vi "RL env test - SAC.vi"() -> ()   [LabVIEW 2024]
uses:
  <vilib>/express/express arith-compare/Formula/XNode/ExpressFormulaBlockNode.xnode
  <vilib>/Analysis/NI_AALBase.lvlib
  <vilib>/measure/NI_MABase.lvlib
panel:
  out "total step":i32
  in  "幅值 2":dbl=1.0
  out "P":dbl(graph)=0.010526704867227326
  out "I":dbl(graph)=1.1597992766160083e-129
  out "start value":dbl[](array[numeric])=[-0.9724784126247488, -0.972476948667373, -0.9724754846716054, -0.9724740206374459, -0.9724725565648947, -0.9724710924539519, -0.9724696283046174, -0.9724681641168914, -0.9724666998907738, -0.9724652356262649, -0.9724637713233645, -0.9724623069820728, -0.9724608426023899, -0.9724593781843156, -0.9724579137278503, -0.9724564492329938, -0.9724549846997463, -0.9724535201281078, -0.9724520555180785, -0.9724505908696581, -0.9724491261828471, -0.9724476614576453, -0.9724461966940527, -0.9724447318920696, -0.9724432670516958, -0.9724418021729316, -0.9724403372557768, -0.9724388723002317, -0.9724374073062962, -0.9724359422739705, -0.9724344772032545, -0.9724330120941482, -0.972431546946652, -0.9724300817607656, -0.9724286165364893, -0.972427151273823, -0.9724256859727668, -0.9724242206333208, -0.972422755255485, -0.9724212898392596, -0.9724198243846445, -0.9724183588916397, -0.9724168933602455, -0.9724154277904618, -0.9724139621822886, -0.972412496535726, -0.9724110308507742, -0.972409565127433, -0.9724080993657028, -0.9724066335655833, -0.9724051677270749, -0.9724037018501773, -0.9724022359348908, -0.9724007699812155, -0.9723993039891512, -0.9723978379586983, -0.9723963718898565, -0.9723949057826261, -0.9723934396370071, -0.9723919734529995, -0.9723905072306035, -0.9723890409698189, -0.9723875746706461, -0.9723861083330848, -0.9723846419571354, -0.9723831755427976, -0.9723817090900718, -0.9723802425989578, -0.972378776069456, -0.972377309501566, -0.9723758428952882, -0.9723743762506224, -0.972372909567569, -0.9723714428461276, -0.9723699760862988, -0.9723685092880822, -0.9723670424514781, -0.9723655755764864, -0.9723641086631073, -0.9723626417113408, -0.972361174721187, -0.9723597076926458, -0.9723582406257175, -0.972356773520402, -0.9723553063766994, -0.9723538391946097, -0.9723523719741332, -0.9723509047152695, -0.9723494374180192, -0.9723479700823818, -0.9723465027083579, -0.9723450352959471, -0.9723435678451497, -0.9723421003559657, -0.9723406328283953, -0.9723391652624382, -0.972337697658095, -0.9723362300153652, -0.9723347623342492, -0.9723332946147469, -0.9723318268568585, -0.972330359060584, -0.9723288912259233, -0.9723274233528767, -0.9723259554414441, -0.9723244874916256, -0.9723230195034213, -0.9723215514768312, -0.9723200834118554, -0.972318615308494, -0.9723171471667469, -0.9723156789866143, -0.9723142107680962, -0.9723127425111927, -0.9723112742159038, -0.9723098058822296, -0.9723083375101702, -0.9723068690997255, -0.9723054006508958, -0.9723039321636809, -0.972302463638081, -0.9723009950740963, -0.9722995264717265, -0.972298057830972, -0.9722965891518325, -0.9722951204343085, -0.9722936516783997, -0.9722921828841063, -0.9722907140514283, -0.972289245180366, -0.972287776270919, -0.9722863073230879, -0.9722848383368722, -0.9722833693122724, -0.9722819002492883, -0.9722804311479202, -0.9722789620081678, -0.9722774928300315, -0.9722760236135111, -0.972274554358607, -0.9722730850653187, -0.972271615733647, -0.9722701463635912, -0.972268676955152, -0.972267207508329, -0.9722657380231224, -0.9722642684995324, -0.9722627989375588, -0.972261329337202, -0.9722598596984617, -0.9722583900213382, -0.9722569203058314, -0.9722554505519415, -0.9722539807596685, -0.9722525109290124, -0.9722510410599734, -0.9722495711525514, -0.9722481012067465, -0.9722466312225588, -0.9722451611999884, -0.9722436911390353, -0.9722422210396995, -0.9722407509019811, -0.9722392807258802, -0.9722378105113969, -0.972236340258531, -0.972234869967283, -0.9722333996376524, -0.97223192926964, -0.972230458863245, -0.9722289884184682, -0.972227517935309, -0.9722260474137682, -0.972224576853845, -0.9722231062555403, -0.9722216356188534, -0.9722201649437852, -0.9722186942303348, -0.9722172234785031, -0.9722157526882895, -0.9722142818596947, -0.9722128109927182, -0.9722113400873604, -0.9722098691436211, -0.9722083981615006, -0.9722069271409988, -0.9722054560821158, -0.9722039849848517, -0.9722025138492065, -0.9722010426751804, -0.9721995714627731, -0.9721981002119852, -0.9721966289228162, -0.9721951575952665, -0.9721936862293361, -0.972192214825025, -0.9721907433823334, -0.9721892719012611, -0.9721878003818084, -0.9721863288239753, -0.9721848572277617, -0.9721833855931679, -0.9721819139201937, -0.9721804422088394, -0.9721789704591048, -0.9721774986709903, -0.9721760268444957, -0.9721745549796211, -0.9721730830763666, -0.9721716111347323, -0.9721701391547182, -0.9721686671363242, -0.9721671950795507, -0.9721657229843975, -0.9721642508508648, -0.9721627786789525, -0.9721613064686608, -0.9721598342199897, -0.9721583619329394, -0.9721568896075097, -0.9721554172437008, -0.9721539448415127, -0.9721524724009456, -0.9721509999219994, -0.9721495274046742, -0.97214805484897, -0.9721465822548871, -0.9721451096224253, -0.9721436369515848, -0.9721421642423655, -0.9721406914947677, -0.9721392187087913, -0.9721377458844362, -0.9721362730217029, -0.972134800120591, -0.9721333271811009, -0.9721318542032323, -0.9721303811869858, -0.9721289081323609, -0.972127435039358, -0.9721259619079768, -0.9721244887382179, -0.9721230155300808, -0.9721215422835661, -0.9721200689986734, -0.972118595675403, -0.9721171223137549, -0.9721156489137291, -0.9721141754753259, -0.9721127019985449, -0.9721112284833866, -0.9721097549298509, -0.9721082813379377, -0.9721068077076473, -0.9721053340389797, -0.9721038603319349, -0.9721023865865129, -0.9721009128027139, -0.9720994389805379, -0.9720979651199849, -0.972096491221055, -0.9720950172837484, -0.9720935433080649, -0.9720920692940047, -0.9720905952415678, -0.9720891211507544, -0.9720876470215645, -0.972086172853998, -0.9720846986480551, -0.9720832244037358, -0.9720817501210404, -0.9720802757999685, -0.9720788014405206, -0.9720773270426963, -0.9720758526064963, -0.9720743781319199, -0.9720729036189679, -0.9720714290676397, -0.972069954477936, -0.972068479849856, -0.9720670051834008, -0.9720655304785695, -0.972064055735363, -0.9720625809537805, -0.972061106133823, -0.9720596312754896, -0.9720581563787812, -0.9720566814436972, -0.9720552064702382, -0.9720537314584037, -0.9720522564081945, -0.9720507813196096, -0.9720493061926503, -0.9720478310273155, -0.9720463558236063, -0.9720448805815217, -0.9720434053010629, -0.9720419299822287, -0.9720404546250205, -0.972038979229437, -0.9720375037954797, -0.9720360283231472, -0.9720345528124409, -0.9720330772633595, -0.9720316016759045, -0.9720301260500745, -0.972028650385871, -0.9720271746832927, -0.9720256989423409, -0.9720242231630145, -0.9720227473453147, -0.9720212714892403, -0.9720197955947928, -0.9720183196619707, -0.9720168436907757, -0.9720153676812061, -0.9720138916332638, -0.9720124155469471, -0.9720109394222577, -0.9720094632591939, -0.9720079870577577, -0.9720065108179472, -0.9720050345397644, -0.9720035582232074, -0.9720020818682782, -0.9720006054749749, -0.9719991290432995, -0.9719976525732502, -0.971996176064829, -0.9719946995180339, -0.9719932229328669, -0.9719917463093263, -0.9719902696474139, -0.9719887929471279, -0.9719873162084702, -0.9719858394314392, -0.9719843626160365, -0.9719828857622607, -0.9719814088701132, -0.9719799319395928, -0.9719784549707007, -0.9719769779634359, -0.9719755009177995, -0.9719740238337905, -0.9719725467114101, -0.9719710695506572, -0.9719695923515329, -0.9719681151140364, -0.9719666378381685, -0.9719651605239285, -0.9719636831713173, -0.971962205780334, -0.9719607283509797, -0.9719592508832534, -0.9719577733771562, -0.9719562958326872, -0.9719548182498473, -0.9719533406286357, -0.9719518629690534, -0.9719503852710996, -0.9719489075347751, -0.9719474297600792, -0.9719459519470128, -0.971944474095575, -0.971942996205767, -0.9719415182775876, -0.971940040311038, -0.9719385623061172, -0.9719370842628263, -0.9719356061811645, -0.9719341280611326, -0.9719326499027298, -0.9719311717059571, -0.9719296934708136, -0.9719282151973004, -0.9719267368854165, -0.971925258535163, -0.9719237801465389, -0.9719223017195453, -0.9719208232541813, -0.9719193447504477, -0.971917866208344, -0.9719163876278708, -0.9719149090090276, -0.971913430351815, -0.9719119516562326, -0.9719104729222808, -0.9719089941499593, -0.9719075153392687, -0.9719060364902085, -0.971904557602779, -0.9719030786769803, -0.9719015997128124, -0.9719001207102754, -0.9718986416693692, -0.9718971625900942, -0.9718956834724499, -0.971894204316437, -0.971892725122055, -0.9718912458893045, -0.971889766618185, -0.9718882873086971, -0.9718868079608404, -0.9718853285746153, -0.9718838491500215, -0.9718823696870594, -0.9718808901857288, -0.9718794106460301, -0.9718779310679628, -0.9718764514515277, -0.9718749717967241, -0.9718734921035527, -0.971872012372013, -0.9718705326021055, -0.9718690527938301, -0.9718675729471868, -0.9718660930621756, -0.9718646131387969, -0.9718631331770503, -0.9718616531769363, -0.9718601731384545, -0.9718586930616054, -0.9718572129463887, -0.9718557327928048, -0.9718542526008533, -0.9718527723705349, -0.971851292101849, -0.9718498117947961, -0.9718483314493759, -0.971846851065589, -0.9718453706434347, -0.971843890182914, -0.9718424096840259, -0.9718409291467714, -0.9718394485711499, -0.971837967957162, -0.9718364873048071, -0.9718350066140861, -0.971833525884998, -0.9718320451175441, -0.9718305643117232, -0.9718290834675365, -0.971827602584983, -0.9718261216640638, -0.971824640704778, -0.9718231597071265, -0.9718216786711086, -0.9718201975967251, -0.9718187164839752, -0.97181723533286, -0.9718157541433784, -0.9718142729155317, -0.9718127916493186, -0.9718113103447406, -0.9718098290017962, -0.9718083476204872, -0.9718068662008119, -0.9718053847427719, -0.9718039032463659, -0.9718024217115953, -0.9718009401384589, -0.9717994585269578, -0.9717979768770911, -0.9717964951888599, -0.9717950134622632, -0.9717935316973021, -0.9717920498939755, -0.9717905680522848, -0.9717890861722286, -0.9717876042538085, -0.9717861222970229, -0.9717846403018736, -0.9717831582683589, -0.9717816761964806, -0.9717801940862371, -0.97177871193763, -0.9717772297506578, -0.9717757475253223, -0.9717742652616217, -0.9717727829595578, -0.9717713006191291, -0.9717698182403373, -0.9717683358231806, -0.9717668533676609, -0.9717653708737766, -0.9717638883415293, -0.9717624057709174, -0.9717609231619428, -0.9717594405146038, -0.9717579578289021, -0.9717564751048361, -0.9717549923424075, -0.9717535095416148, -0.9717520267024594, -0.9717505438249402, -0.9717490609090584, -0.9717475779548129, -0.971746094962205, -0.9717446119312335, -0.9717431288618996, -0.9717416457542023, -0.9717401626081427, -0.9717386794237198, -0.9717371962009347, -0.9717357129397864, -0.9717342296402761, -0.9717327463024028, -0.9717312629261674, -0.9717297795115692, -0.9717282960586091, -0.9717268125672862, -0.9717253290376016, -0.9717238454695543, -0.9717223618631453, -0.9717208782183738, -0.9717193945352408, -0.9717179108137454, -0.9717164270538886, -0.9717149432556694, -0.971713459419089, -0.9717119755441463, -0.9717104916308427, -0.9717090076791767, -0.9717075236891499, -0.9717060396607609, -0.9717045555940113, -0.9717030714888995, -0.9717015873454271, -0.9717001031635928, -0.971698618943398, -0.9716971346848414, -0.9716956503879245, -0.9716941660526458, -0.9716926816790069, -0.9716911972670064, -0.9716897128166457, -0.9716882283279236, -0.9716867438008415, -0.971685259235398, -0.9716837746315946, -0.97168228998943, -0.9716808053089055, -0.97167932059002, -0.9716778358327749, -0.9716763510371687, -0.971674866203203, -0.9716733813308763, -0.9716718964201904, -0.9716704114711435, -0.9716689264837375, -0.9716674414579707, -0.9716659563938448, -0.9716644712913582, -0.9716629861505127, -0.9716615009713067, -0.9716600157537418, -0.9716585304978165, -0.9716570452035325, -0.9716555598708881, -0.9716540744998852, -0.9716525890905221, -0.9716511036428004, -0.9716496181567188, -0.9716481326322787, -0.9716466470694788, -0.9716451614683205, -0.9716436758288024, -0.9716421901509261, -0.9716407044346902, -0.9716392186800963, -0.9716377328871427, -0.9716362470558313, -0.9716347611861603, -0.9716332752781316, -0.9716317893317435, -0.9716303033469977, -0.9716288173238928, -0.9716273312624302, -0.9716258451626086, -0.9716243590244295, -0.9716228728478914, -0.9716213866329959, -0.9716199003797417, -0.9716184140881301, -0.9716169277581599, -0.9716154413898325, -0.9716139549831465, -0.9716124685381035, -0.971610982054702, -0.9716094955329435, -0.9716080089728268, -0.9716065223743532, -0.9716050357375214, -0.9716035490623329, -0.9716020623487863, -0.9716005755968832, -0.9715990888066219, -0.9715976019780044, -0.9715961151110288, -0.9715946282056971, -0.9715931412620074, -0.9715916542799616, -0.971590167259558, -0.9715886802007986, -0.9715871931036814, -0.9715857059682085, -0.9715842187943778, -0.9715827315821917, -0.9715812443316478, -0.9715797570427487, -0.9715782697154919, -0.97157678234988, -0.9715752949459104, -0.971573807503586, -0.9715723200229041, -0.9715708325038672, -0.9715693449464731, -0.9715678573507242, -0.971566369716618, -0.9715648820441573, -0.9715633943333394, -0.971561906584167, -0.9715604187966376, -0.9715589309707537, -0.971557443106513, -0.9715559552039181, -0.9715544672629663, -0.9715529792836605, -0.9715514912659979, -0.9715500032099813, -0.9715485151156082, -0.9715470269828812, -0.9715455388117977, -0.9715440506023605, -0.9715425623545669, -0.9715410740684197, -0.9715395857439163, -0.9715380973810593, -0.9715366089798463, -0.9715351205402798, -0.9715336320623573, -0.9715321435460815, -0.97153065499145, -0.9715291663984651, -0.9715276777671246, -0.9715261890974309, -0.9715247003893817, -0.9715232116429795, -0.9715217228582218, -0.9715202340351112, -0.9715187451736453, -0.9715172562738267, -0.9715157673356528, -0.9715142783591263, -0.9715127893442447, -0.9715113002910105, -0.9715098111994214, -0.9715083220694798, -0.9715068329011833, -0.9715053436945347, -0.9715038544495311, -0.9715023651661755, -0.9715008758444652, -0.9714993864844028, -0.971497897085986, -0.9714964076492172, -0.971494918174094, -0.9714934286606189, -0.9714919391087896, -0.9714904495186086, -0.9714889598900734, -0.9714874702231867, -0.9714859805179459, -0.9714844907743536, -0.9714830009924074, -0.9714815111721098, -0.9714800213134585, -0.9714785314164558, -0.9714770414810995, -0.9714755515073921, -0.971474061495331, -0.971472571444919, -0.9714710813561536, -0.9714695912290372, -0.9714681010635675, -0.9714666108597471, -0.9714651206175734, -0.9714636303370491, -0.9714621400181717, -0.9714606496609437, -0.9714591592653627, -0.9714576688314314, -0.9714561783591472, -0.9714546878485126, -0.9714531972995254, -0.971451706712188, -0.9714502160864978, -0.9714487254224577, -0.971447234720065, -0.9714457439793225, -0.9714442532002274, -0.9714427623827827, -0.9714412715269855, -0.9714397806328388, -0.9714382897003396, -0.9714367987294912, -0.9714353077202904, -0.9714338166727405, -0.9714323255868383, -0.9714308344625872, -0.9714293432999838, -0.9714278520990316, -0.9714263608597272, -0.9714248695820743, -0.9714233782660692, -0.9714218869117157, -0.9714203955190102, -0.9714189040879564, -0.9714174126185505, -0.9714159211107967, -0.9714144295646908, -0.9714129379802371, -0.9714114463574315, -0.9714099546962781, -0.9714084629967731, -0.9714069712589203, -0.9714054794827159, -0.9714039876681639, -0.9714024958152606, -0.9714010039240096, -0.9713995119944075, -0.9713980200264579, -0.9713965280201572, -0.9713950359755091, -0.9713935438925101, -0.9713920517711638, -0.9713905596114667, -0.9713890674134225, -0.9713875751770275, -0.9713860829022855, -0.9713845905891928, -0.9713830982377533, -0.9713816058479632, -0.9713801134198264, -0.9713786209533392, -0.9713771284485054, -0.9713756359053212, -0.9713741433237907, -0.9713726507039097, -0.9713711580456826, -0.9713696653491052, -0.9713681726141818, -0.9713666798409082, -0.9713651870292888, -0.9713636941793191, -0.9713622012910038, -0.9713607083643384, -0.9713592153993275, -0.9713577223959665, -0.9713562293542602, -0.971354736274204, -0.9713532431558026, -0.9713517499990513, -0.971350256803955, -0.9713487635705088, -0.9713472702987179, -0.9713457769885772, -0.9713442836400918, -0.9713427902532568, -0.9713412968280771, -0.971339803364548, -0.9713383098626744, -0.9713368163224514, -0.9713353227438841, -0.9713338291269674, -0.9713323354717066, -0.9713308417780966, -0.9713293480461425, -0.9713278542758393, -0.9713263604671921, -0.9713248666201961, -0.9713233727348561, -0.9713218788111675, -0.9713203848491349, -0.9713188908487538, -0.9713173968100288, -0.9713159027329555, -0.9713144086175385, -0.9713129144637732, -0.9713114202716644, -0.9713099260412074, -0.9713084317724069, -0.9713069374652584, -0.9713054431197665, -0.9713039487359268, -0.9713024543137437, -0.9713009598532131, -0.9712994653543391, -0.9712979708171176, -0.9712964762415529, -0.9712949816276408, -0.9712934869753858, -0.9712919922847834, -0.9712904975558381, -0.9712890027885456, -0.9712875079829103, -0.971286013138928, -0.971284518256603, -0.9712830233359311, -0.9712815283769166, -0.9712800333795553, -0.9712785383438516, -0.9712770432698011, -0.9712755481574084, -0.971274053006669, -0.9712725578175875, -0.9712710625901595, -0.9712695673243894, -0.971268072020273, -0.9712665766778146, -0.97126508129701, -0.9712635858778634, -0.9712620904203709, -0.9712605949245365, -0.9712590993903563, -0.9712576038178343, -0.9712561082069665, -0.9712546125577572, -0.9712531168702022, -0.9712516211443057, -0.9712501253800637, -0.9712486295774804, -0.9712471337365516, -0.9712456378572816, -0.9712441419396662, -0.9712426459837098, -0.9712411499894081, -0.9712396539567655, -0.9712381578857778, -0.9712366617764492, -0.9712351656287758, -0.9712336694427613, -0.9712321732184024, -0.9712306769557024, -0.9712291806546581, -0.971227684315273, -0.9712261879375435, -0.9712246915214733, -0.9712231950670589, -0.971221698574304, -0.9712202020432049, -0.9712187054737655, -0.9712172088659821, -0.9712157122198584, -0.9712142155353907, -0.971212718812583, -0.9712112220514313, -0.9712097252519398, -0.9712082284141044, -0.9712067315379294, -0.9712052346234105, -0.971203737670552, -0.9712022406793499, -0.9712007436498084, -0.9711992465819232, -0.9711977494756988, -0.9711962523311309, -0.9711947551482238, -0.9711932579269735, -0.971191760667384, -0.9711902633694514, -0.9711887660331797, -0.971187268658565, -0.9711857712456115, -0.9711842737943148, -0.9711827763046796, -0.9711812787767015, -0.9711797812103848, -0.9711782836057253, -0.9711767859627275, -0.9711752882813869, -0.971173790561708, -0.9711722928036866, -0.971170795007327, -0.9711692971726248, -0.9711677992995847, -0.9711663013882021, -0.9711648034384818, -0.9711633054504191, -0.9711618074240187, -0.971160309359276, -0.9711588112561959, -0.9711573131147735, -0.9711558149350138, -0.971154316716912, -0.971152818460473, -0.971151320165692, -0.9711498218325738, -0.9711483234611138, -0.9711468250513168, -0.971145326603178, -0.9711438281167024, -0.9711423295918851, -0.9711408310287312, -0.9711393324272355, -0.9711378337874035, -0.9711363351092298, -0.9711348363927199, -0.9711333376378684, -0.9711318388446808, -0.9711303400131517, -0.9711288411432867, -0.9711273422350802, -0.9711258432885381, -0.9711243443036546, -0.9711228452804355, -0.9711213462188751, -0.9711198471189793, -0.9711183479807423, -0.9711168488041699, -0.9711153495892566, -0.9711138503360079, -0.9711123510444185, -0.9711108517144939, -0.9711093523462285, -0.9711078529396281, -0.9711063534946871, -0.9711048540114111, -0.9711033544897947, -0.9711018549298434, -0.9711003553315518, -0.9710988556949254, -0.971097356019959, -0.9710958563066576, -0.9710943565550165, -0.9710928567650405, -0.971091356936725, -0.9710898570700747, -0.9710883571650849, -0.9710868572217604, -0.9710853572400966, -0.9710838572200982, -0.9710823571617607, -0.9710808570650886, -0.9710793569300776, -0.9710778567567321, -0.9710763565450479, -0.9710748562950291, -0.9710733560066719, -0.9710718556799801, -0.9710703553149501, -0.9710688549115856, -0.971067354469883, -0.971065853989846, -0.9710643534714711, -0.9710628529147619, -0.9710613523197149, -0.9710598516863337, -0.9710583510146148, -0.9710568503045618, -0.9710553495561713, -0.9710538487694468, -0.971052347944385, -0.9710508470809891, -0.9710493461792562, -0.9710478452391892, -0.9710463442607854, -0.9710448432440476, -0.9710433421889731, -0.9710418410955648, -0.9710403399638199, -0.9710388387937412, -0.9710373375853261, -0.9710358363385773, -0.9710343350534921, -0.9710328337300734, -0.9710313323683186, -0.9710298309682303, -0.971028329529806, -0.9710268280530482, -0.9710253265379547, -0.9710238249845278, -0.9710223233927653, -0.9710208217626694, -0.9710193200942381, -0.9710178183874735, -0.9710163166423736, -0.9710148148589407, -0.9710133130371725, -0.9710118111770714, -0.9710103092786351, -0.971008807341866, -0.9710073053667618, -0.9710058033533251, -0.9710043013015532, -0.971002799211449, -0.9710012970830099, -0.9709997949162384, -0.9709982927111321, -0.9709967904676936]
  out "I":dbl=1.1597992766160083e-129
  out "P":dbl=0.010526704867227326
  out "ZVolt":dbl(graph)=0.314
  out "largest reward episode":picture
  out "initialized array":dbl[](array[numeric])
  out "ep reward":dbl(graph)=11.830070995768676
  out "loss_c":dbl(graph)=1731497.5
  out "loss_a":dbl(graph)=6725.31298828125
  out "max ep reward":dbl=24543.99785734303
  out "batch_size":i32=256
  in  "base batch number":i32=256
  out "ep reward":dbl=3677.849231856129
  out "PIDoutput":dbl=0.0008497199147603398
  out "Reward":dbl=4.912643239900043
  out "errorsum":dbl=-0.005069024381114479
  out "ZVolt":dbl=0.129
  out "return value":dbl[](array[numeric])=[0.128, -0.005028664176972831, 0.0008485916053116275, 4.912763807403283, 5000.08984375, 122631.6953125, 0.01052668650438312, 1.663726715006467e-129, 30902.0]
  out "loss_c":dbl=23912.59765625
  out "loss_a":dbl=4978.1279296875
  out "ep loop":i32=506
  out "topo":dbl[][](array[numeric])
  in  "扫描像素":i32=500
  in  "deflection setpoint\nV":dbl=0.5 caption="defl setpoint\n/V" format="%.2f"
  in  "spring constant\nN/m":dbl=2.34
  in  "invOLS\nm/V":dbl=1e-07
  in  "noise amp":dbl caption="noise 幅值" format="%0.2f"
  out "tem topo":dbl[](array[numeric])=[187.7613450258975, 187.61388643049506, 187.4625946204324, 187.30747590277633, 187.14853587042907, 186.98578082132366, 186.81921706928887, 186.64885137876908, 186.4746905808606, 186.29674199265563, 186.1150123695872, 185.92950817277307, 185.74023679128615, 185.5472059277571, 185.3504235460163, 185.14989781279343, 184.94563633899963, 184.7376469430854, 184.52593768641884, 184.3105160636524, 184.09139078628462, 183.86857162664072, 183.64206782984775, 183.41188762880165, 183.17803969715476, 182.940533253404, 182.6993776738212, 182.45458275299467, 182.2061581201141, 181.9541137790551, 181.69845902351616, 181.4392040047092, 181.17635923335035, 180.9099353647009, 180.63994279021992, 180.36639272167008, 180.0892956631369, 179.80866218898547, 179.52450272102482, 179.23682835570867, 178.9456510293229, 178.6509823562041, 178.35283451751783, 178.05121924067203, 177.74614789904152, 177.43763209086856, 177.1256831579414, 176.81031438615872, 176.49153920701886, 176.1693704250344, 175.8438197839498, 175.5148992710352, 175.1826220036406, 174.84700179662502, 174.50805226675456, 174.1657866700021, 173.82021882777377, 173.4713618312618, 173.11922905760952, 172.76383369071877, 172.40519035359426, 172.04331373418668, 171.67821862608477, 171.309919247784, 170.93842996746667, 170.56376459454503, 170.1859381629234, 169.80496661154504, 169.42086450264173, 169.0336461495204, 168.64332644908936, 168.24992153572245, 167.8534472210812, 167.45391914002545, 167.05135290786737, 166.64576477592976, 166.23717056004534, 165.8255864580667, 165.41102824418462, 164.993512051037, 164.5730539824388, 164.14967149000674, 163.72338154946098, 163.29420163843847, 162.8621478997749, 162.42723600545892, 161.98948326866116, 161.54890821264763, 161.10552891654612, 160.65936182203373, 160.2104244383099, 159.75873339582176, 159.30430783151849, 158.84716617980712, 158.38732582179352, 157.92480465368322, 157.45962095462795, 156.9917931204645, 156.52134079311634, 156.04828181301244, 155.5726339452858, 155.09441638968062, 154.6136472489628, 154.13034603381615, 153.64453342334664, 153.15622823962474, 152.6654487644259, 152.17221427862043, 151.67654406165875, 151.17845773475776, 150.6779754198373, 150.1751166395368, 149.6699009678266, 149.16234857689454, 148.65247965734684, 148.14031472217746, 147.6258735036707, 147.10917499961235, 146.59023960513701, 146.06908936048072, 145.54574534752848, 145.0202280189793, 144.49255697285886, 143.9627528409633, 143.43083662447464, 142.89683103403888, 142.36075609849416, 141.8226322377577, 141.28248084096668, 140.7403228358143, 140.19618147026964, 139.65007719448658, 139.10203138144058, 138.5520648385552, 138.0001998189378, 137.44645916616463, 136.8908646299422, 136.33343835957476, 135.77420029905568, 135.2131729773161, 134.65037927199438, 134.085842517716, 133.51958398463665, 132.95162590146327, 132.38198951126483, 131.81069772747327, 131.23777582486153, 130.66324602136686, 130.08712810940673, 129.50944270227356, 128.9302148852338, 128.34946995048892, 127.76723132900268, 127.1835223957668, 126.59836313273254, 126.0117743805774, 125.42378171891849, 124.83440802553078, 124.24367865056477, 123.65161705267003, 123.05824537033818, 122.46358737016546, 121.8676660763033, 121.27050397839896, 120.67212509303626, 120.07255452365224, 119.47181429525949, 118.86992771340098, 118.26691945109958, 117.66281486922844, 117.05763699983594, 116.45140914898187, 115.84415486761131, 115.23589739677422, 114.62666129469993, 114.01647170371834, 113.4053523678418, 112.79332761724639, 112.18042094737417, 111.56665539163178, 110.95205657012772, 110.33664908843807, 109.7204567805789, 109.10350337562569, 108.48581429969163, 107.86741457937245, 107.24832916589155, 106.62858082996027, 106.00819263635799, 105.38718869341413, 104.76559399003862, 104.1434364037364, 103.52074069435302, 102.89752945766561, 102.27382523581976, 101.64965224143607, 101.0250378083464, 100.4000075640133, 99.77458579919268, 99.1487949153723, 98.52265906971381, 97.89620440697074, 97.26945584154277, 96.64244000241739, 96.01518209293741, 95.38770529956422, 94.76003198981391, 94.13218671610107, 93.50419571582589, 92.87608519661319, 92.24788071347997, 91.61960554934515, 90.99128322185149, 90.36293885140294, 89.73459833622178, 89.10628770918771, 88.47803030643058, 87.84985008435751, 87.22177373506835, 86.59382458272312, 85.96602876753649, 85.33841005320626, 84.71099133420107, 84.08379740659025, 83.45685581207407, 82.83019160660528, 82.20382991407092, 81.57779526064273, 80.95210936674015, 80.32679554916554, 79.70188178789725, 79.07739412234078, 78.45335970976134, 77.82979964411959, 77.2067353165578, 76.5841915304312, 75.96219562894171, 75.34077282899595, 74.71994845171014, 74.0997464577927, 73.48018780517437, 72.8612969192854, 72.24310150008678, 71.62562695271967, 71.00889694495794, 70.39293416106386, 69.77776243437484]
  in  "frequency 2":dbl=0.001
  in  "amplitude":dbl caption="幅值 1" format="%0.2p"
  in  "effective\nmodulus\nPa":dbl=1500000000.0
  in  "tip\nradius\nnm":dbl=1e-08
  in  "a0\nnm 2":dbl=4e-10
  in  "hamaker\nconstant":dbl=4.25e-19
  out "Fs":dbl=1000.0
  out "error":dbl(graph)=0.0806133634699095
  out "#s":dbl=1000.0
  in  "sampling info":cluster{"Fs":dbl, "#s":dbl}={"Fs"=1000.0, "#s"=1000.0} caption="采样信息" {"Fs" format="%.2p"}
  in  "frequency":dbl=0.01 caption="frequency 1" format="%0.2p"
  out "separation":dbl(graph)=-6.006813032198851e-09
  out "defl voltage":dbl(graph)=0.4193866365300905
  out "control signal":dbl(graph)=0.9638211864355544
  out "sample surface":dbl[][](graph)=[[76.39974719326271, 70.39293416106386]]
  out "done":bool
  out "step loop":i32=747
types:
  T1 = typedef "imagedata.ctl" = cluster{"image type":i32, "image depth":i32, "image":u8[], "mask":u8[], "colors":u32[], "Rectangle":cluster{"left":i16, "top":i16, "right":i16, "bottom":i16}}
  T2 = typedef "NI_Matrix.lvlib/RealMatrix.ctl" = dbl[][]
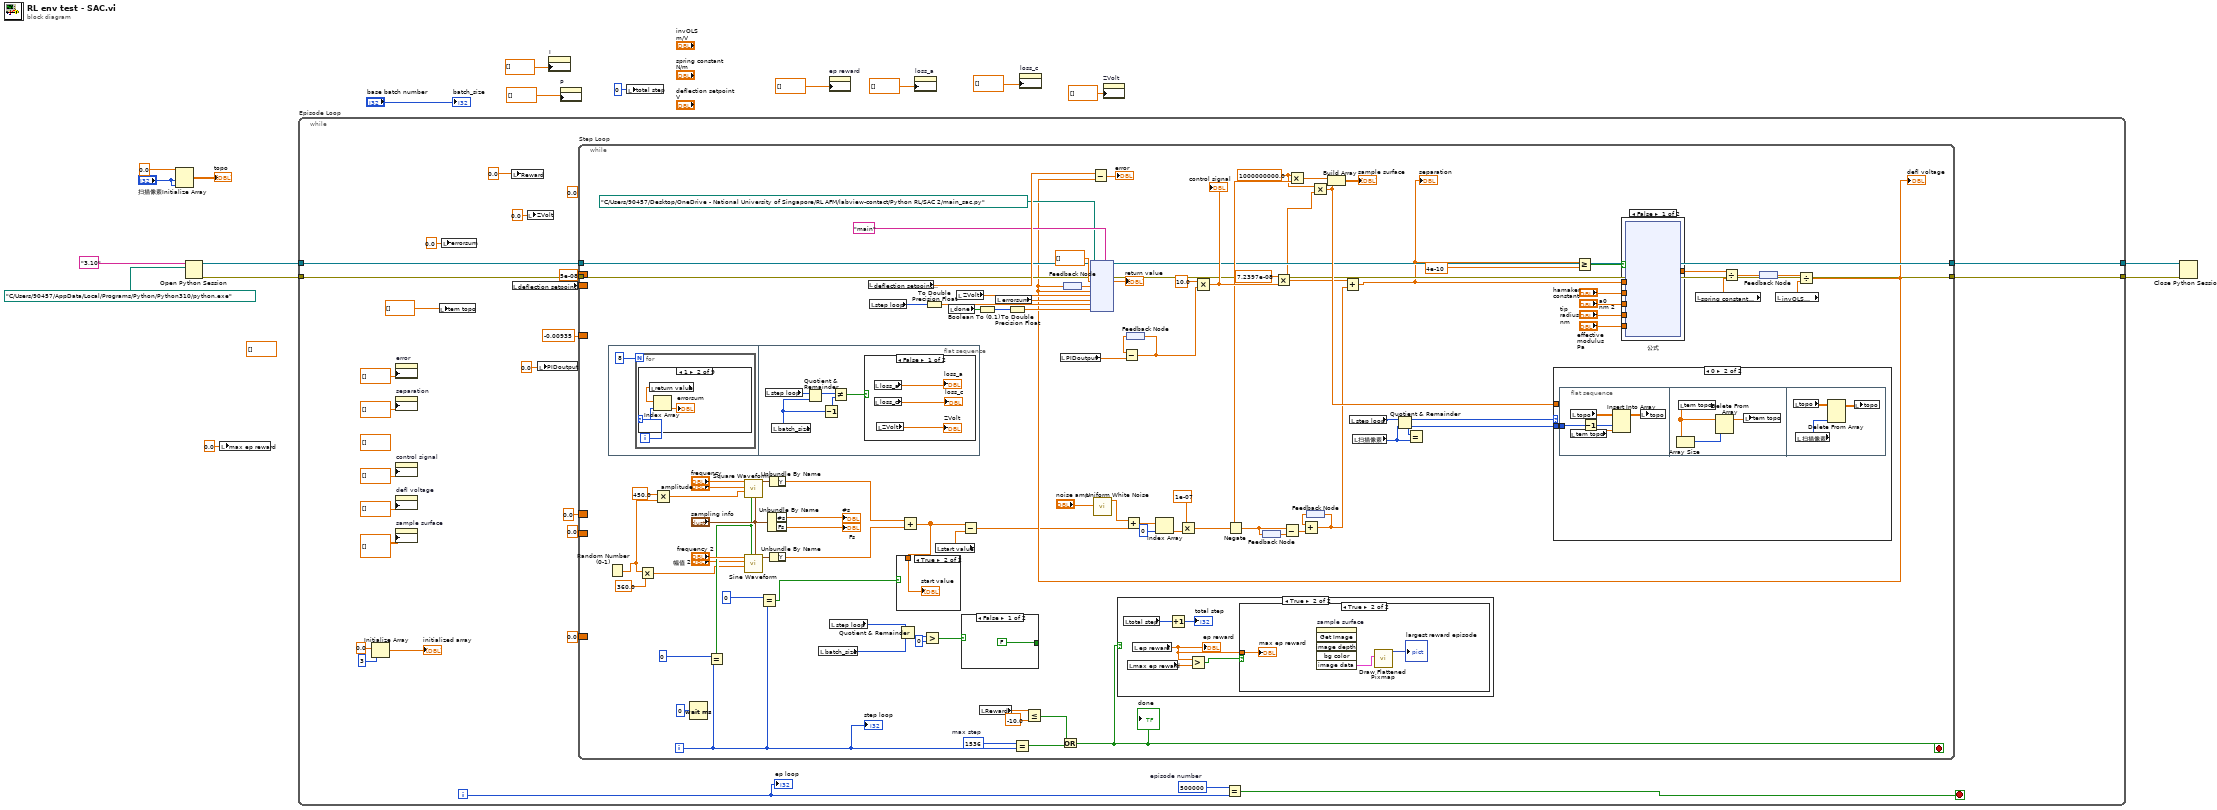
[diagram p0: block diagram]
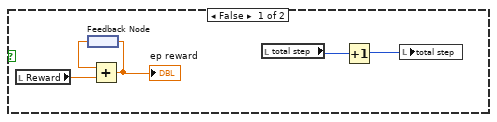
[diagram p3: hidden frame]
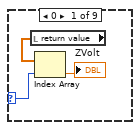
[diagram p5: hidden frame]
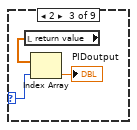
[diagram p6: hidden frame]
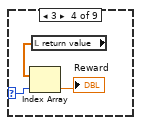
[diagram p7: hidden frame]
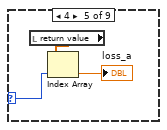
[diagram p8: hidden frame]
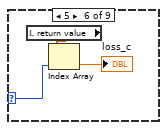
[diagram p9: hidden frame]
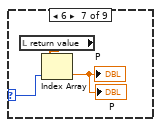
[diagram p10: hidden frame]
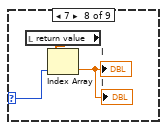
[diagram p11: hidden frame]
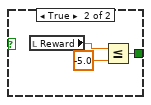
[diagram p14: hidden frame]
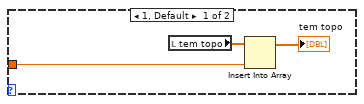
[diagram p15: hidden frame]
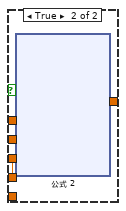
[diagram p16: hidden frame]
diagram:
  (unwired) dbl[] []
  n1 = Initialize Array(0.0 ("元素"), "扫描像素", "扫描像素") -> (→"topo":dbl[][])
  n2 = Open Python Session(python version="3.10" ("Python version"), python path=path "C:/Users/90457/AppData/Local/Programs/Python/Python310/python.exe" ("Python path")) -> (session out=w15:refnum<k35>, error out=w14:errorcluster)  [unwired: 1 in]
  n3 = local write "max ep reward"(0.0 ("max ep reward")) -> ()
  n4 = while "Episode Loop" {
    tunnel: w15 -> [w30]
    tunnel: w14 -> [w29]
    tunnel: [w28] -> w11
    tunnel: [w27] -> w10
    i -> [w40]
    stop <- w44 stop-if-true
    (unwired) 0.0
    (unwired) dbl[] [] ("History Data")
    w32 = 500000  # episode number
    n5 = Initialize Array(0.0 ("element"), 3 ("dimension size")) -> (→"initialized array":dbl[])
    n6 = property on="error" class="WFChart (strict)"("History Data"=dbl[] []) -> ()  [unwired: 2 in, 2 out]
    n7 = property on="separation" class="WFChart (strict)"("History Data"=dbl[] []) -> ()  [unwired: 2 in, 2 out]
    n8 = property on="control signal" class="WFChart (strict)"("History Data"=dbl[] []) -> ()  [unwired: 2 in, 2 out]
    n9 = property on="defl voltage" class="WFChart (strict)"("History Data"=dbl[] []) -> ()  [unwired: 2 in, 2 out]
    n10 = property on="sample surface" class="WFChart (strict)"("History Data"=dbl[][] []) -> ()  [unwired: 2 in, 2 out]
    n11 = local write "tem topo"(dbl[] [] ("History Data")) -> ()
    n12 = local write "errorsum"(0.0 ("errorsum")) -> ()
    n13 = local write "Reward"(0.0) -> ()
    n14 = local read "deflection setpoint\nV"() -> (w43:dbl)
    n15 = local write "ZVolt"(0.0 ("ZVolt")) -> ()
    n16 = local write "PIDoutput"(0.0 ("PIDoutput")) -> ()
    n17 = while "Step Loop" {
      tunnel: [w94] -> w28
      tunnel: [w68] -> w27
      border: w43 -> [_]
      border: 0.0 -> [_]
      border: 5e-08 -> [_]
      border: 0.0 -> [_]
      tunnel: w30 -> [w72]
      tunnel: w29 -> [w71]
      border: 0.0 -> [_]
      border: -0.00935 -> [_]
      i -> [w64]
      stop <- w73 stop-if-true
      w111 = 1000000000.0 ("x")
      w88 = 1536  # max step
      n18 = flat-sequence {
        frame #0 {
          n19 = for {
            N: 8 -> [_]
            i -> [w154]
            n20 = case shown="1" w154 {
              selector: w154 -> [w157 w160 w161 w166 w169 w172 w174 w177 _]
              frame 0 {
                n21 = local read "return value"() -> (w156:dbl[])
                n22 = Index Array(array=w156, index=w157) -> (element=→"ZVolt":dbl)
              }
              frame 1 {
                n23 = local read "return value"() -> (w159:dbl[])
                n24 = Index Array(array=w159, index=w160) -> (element=→"errorsum":dbl)
              }
              frame 2 {
                n25 = local read "return value"() -> (w163:dbl[])
                n26 = Index Array(array=w163, index=w161) -> (element=→"PIDoutput":dbl)
              }
              frame 3 {
                n27 = local read "return value"() -> (w165:dbl[])
                n28 = Index Array(array=w165, index=w166) -> (element=→"Reward":dbl)
              }
              frame 4 {
                n29 = local read "return value"() -> (w168:dbl[])
                n30 = Index Array(array=w168, index=w169) -> (element=→"loss_a":dbl)
              }
              frame 5 {
                n31 = local read "return value"() -> (w171:dbl[])
                n32 = Index Array(array=w171, index=w172) -> (element=→"loss_c":dbl)
              }
              frame 6 {
                n33 = local read "return value"() -> (w175:dbl[])
                n34 = Index Array(array=w175, index=w174) -> (element=→"P" →"P":dbl)
              }
              frame 7 {
                n35 = local read "return value"() -> (w178:dbl[])
                n36 = Index Array(array=w178, index=w177) -> (element=→"I" →"I":dbl)
              }
              frame 9, Default {
              }
            }
          }
        }
        frame #1 {
          n37 = local read "step loop"() -> (w181:i32)
          n38 = local read "batch_size"() -> (w179:i32)
          n39 = Quotient & Remainder(x=w181, y=w179) -> (x-y*floor(x/y)=w182:i32)  [unwired: 1 out]
          n40 = Decrement(x=w179) -> (x-1=w180:i32)
          n41 = Not Equal?(x=w182, y=w180) -> (x != y?=w183:bool)
          n42 = case shown="False" w183 {
            frame False {
              n43 = local read "loss_a"() -> (→"loss_a":dbl)
              n44 = local read "loss_c"() -> (→"loss_c":dbl)
              n45 = local read "ZVolt"() -> (→"ZVolt":dbl)
            }
            frame True {
            }
          }
        }
      }
      n46 = Random Number (0-1)() -> (number: 0 to 1=w46:dbl)
      n47 = Multiply(x=w46, y=360.0) -> (x*y=w53:dbl)
      n48 = Multiply(x=450.0, y=w46) -> (x*y=w47:dbl)
      n49 = Wait (ms)(milliseconds to wait=u32 0) -> ()  [unwired: 1 out]
      n50 = Equal?(x=0, y=w64) -> (x = y?=w86:bool)
      n51 = call <vilib>:"Square Waveform.vi"("sampling info"="sampling info", "reset signal"=w86, "phase"=w47, "amplitude"="amplitude", "frequency"="frequency") -> ("signal out"=w133:waveform(dbl))  [unwired: 5 in, 1 out]
      n52 = call <vilib>:"Sine Waveform.vi"("sampling info"="sampling info", "reset signal"=w86, "phase"=w53, "amplitude"="幅值 2", "frequency"="frequency 2") -> ("signal out"=w109:waveform(dbl))  [unwired: 5 in, 1 out]
      n53 = Equal?(x=0, y=w64) -> (x = y?=w66:bool)
      n54 = Unbundle By Name("sampling info") -> ("#s"=→"#s":dbl, "Fs"=→"Fs":dbl)
      n55 = Unbundle By Name(w133) -> ("Y"=w101:dbl[])
      n56 = Unbundle By Name(w109) -> ("Y"=w65:dbl[])
      n57 = local read "batch_size"() -> (w69:i32)
      n58 = local read "step loop"() -> (w84:i32)
      n59 = local read "deflection setpoint\nV"() -> (w100:dbl)
      n60 = local read "step loop"() -> (w89:i32)
      n61 = Quotient & Remainder(x=w84, y=w69) -> (floor(x/y)=w83:i32)  [unwired: 1 out]
      n62 = Add(x=w101, y=w65) -> (x+y=w50:dbl[])
      n63 = case shown="True" w66 {
        tunnel: w50 -> [_ w139]
        frame False {
        }
        frame True {
          "start value" <- w139
        }
      }
      n64 = Greater?(x=w83, y=0) -> (0:w81:bool)
      n65 = To Double Precision Float(number=w89) -> (double precision float=w79:dbl)
      n66 = local read "start value"() -> (w52:dbl[])
      n67 = local read "done"() -> (w91:bool)
      n68 = local read "ZVolt"() -> (w74:dbl)
      n69 = case shown="False" w81 {
        tunnel: [FALSE w188] -> _
        frame False {
        }
        frame True {
          n70 = local read "Reward"() -> (w189:dbl)
          n71 = Less Or Equal?(x=w189, y=-5.0) -> (x <= y?=w188:bool)
        }
      }
      n72 = Subtract(x=w50, y=w52) -> (x-y=w51:dbl[])
      n73 = Boolean To (0,1)(Boolean=w91) -> (0, 1=w93:i16)
      n74 = local read "Reward"() -> (w77:dbl)
      n75 = local read "errorsum"() -> (w75:dbl)
      n76 = To Double Precision Float(number=w93) -> (double precision float=w80:dbl)
      n77 = Equal?(x=w88, y=w64) -> (x = y?=w78:bool)
      n78 = Less Or Equal?(x=w77, y=-10.0) -> (x <= y?=w49:bool)
      n79 = local read "PIDoutput"() -> (w57:dbl)
      n80 = Or(x=w49, y=w78) -> (x .or. y?=w73:bool)
      "done" <- w73
      n81 = feedback #1 ("反馈节点")() -> (w95:dbl)
      n82 = call <vilib>:"Uniform White Noise.vi"("amplitude"="noise amp") -> ("uniform white noise"=w103:dbl[])  [unwired: 9 in, 1 out]
      n83 = case shown="True" w73 {
        frame False {
          n84 = local read "Reward"() -> (w144:dbl)
          n85 = feedback #2() -> (w142:dbl)
          n86 = Add(x=w142, y=w144) -> (x+y=w143:dbl)
          "ep reward" <- w143
          n87 = feedback-in #2(w143) -> ()
          n88 = local read "total step"() -> (w141:i32)
          n89 = Increment(x=w141) -> (x+1=w140:i32)
          n90 = local write "total step"(w140) -> ()
        }
        frame True {
          n91 = local read "total step"() -> (w146:i32)
          n92 = local read "max ep reward"() -> (w148:dbl)
          n93 = local read "ep reward"() -> (w147:dbl)
          "ep reward" <- w147
          n94 = Increment(x=w146) -> (x+1=→"total step":i32)
          n95 = Greater?(x=w147, y=w148) -> (0:w149:bool)
          n96 = case shown="True" w149 {
            tunnel: w147 -> [_ w152]
            frame False {
            }
            frame True {
              n97 = invoke on="sample surface" class="WFChart (strict)" method="Get Image"() -> ("image data"=w151:T1)  [unwired: 6 in, 5 out]
              n98 = call <vilib>:"Draw Flattened Pixmap.vi"("image data"=w151) -> ("new picture"=→"largest reward episode":picture)  [unwired: 8 in]
              "max ep reward" <- w152
            }
          }
        }
      }
      n99 = Add(x=w103, y=w51) -> (x+y=w102:dbl[])
      n100 = feedback #3() -> (w56:dbl)
      n101 = Subtract(x=w56, y=w57) -> (x-y=w55:dbl)
      n102 = feedback-in #3(w55) -> ()
      n103 = Index Array(array=w102, index=0 ("索引")) -> (element=w124:dbl)
      n104 = Multiply(x=1e-07, y=w124) -> (x*y=w113:dbl)
      n105 = Multiply(x=10.0, y=w55) -> (x*y=w119:dbl)
      "control signal" <- w119
      n106 = Negate(x=w113) -> (-x=w121:dbl)
      n107 = feedback #4() -> (w122:dbl)
      n108 = feedback-in #4(w121) -> ()
      n109 = Multiply(x=7.2397e-08 ("zp sns"), y=w119) -> (x*y=w58:dbl)
      n110 = Subtract(x=w121, y=w122) -> (x-y=w61:dbl)
      n111 = Multiply(x=w111, y=w113) -> (x*y=w112:dbl)
      n112 = feedback #5() -> (w62:dbl)
      n113 = Add(x=w62, y=w61) -> (x+y=w60:dbl)
      n114 = feedback-in #5(w60) -> ()
      n115 = Multiply(x=w111, y=w58) -> (x*y=w106:dbl)
      n116 = Build Array(w112, w106) -> (→"sample surface":T2)
      n117 = Add(x=w58, y=w60) -> (x+y=w59:dbl)
      "separation" <- w59
      n118 = local read "step loop"() -> (w90:i32)
      n119 = local read "扫描像素"() -> (w99:i32)
      n120 = Quotient & Remainder(x=w90, y=w99) -> (x-y*floor(x/y)=w107:i32, floor(x/y)=w105:i32)
      n121 = Equal?(x=w105, y=w99) -> ()  [unwired: 1 out]
      n122 = case shown="0" w107 {
        tunnel: w106 -> [w193 _]
        tunnel: w105 -> [_ w194]
        frame 1, Default {
          n123 = local read "tem topo"() -> (w191:dbl[])
          n124 = Insert Into Array(array=w191, new element=w193) -> (→"tem topo":dbl[])  [unwired: 1 in]
        }
        frame 0 {
          n125 = flat-sequence {
            tunnel: w194 -> [w196]
            frame #0 {
              n126 = local read "tem topo"() -> (w199:dbl[])
              n127 = local read "topo"() -> (w195:dbl[][])
              n128 = Decrement(x=w196) -> (x-1=w197:i32)
              n129 = Insert Into Array(array=w195, index (col)=w197, new element=w199) -> (w198:dbl[][])  [unwired: 1 in]
              n130 = local write "topo"(w198) -> ()
            }
            frame #1 {
              n131 = local read "tem topo"() -> (w202:dbl[])
              n132 = Array Size(array=w202) -> (size(s)=w201:i32)
              n133 = Delete From Array(array=w202, length=w201) -> (array with subset deleted=w200:dbl[])  [unwired: 1 in, 1 out]
              n134 = local write "tem topo"(w200) -> ()
            }
            frame #2 {
              n135 = local read "topo"() -> (w205:dbl[][])
              n136 = local read "扫描像素"() -> (w204:i32)
              n137 = Delete From Array(array=w205, index (col)=w204) -> (array with subset deleted=w203:dbl[][])  [unwired: 2 in, 1 out]
              n138 = local write "topo"(w203) -> ()
            }
          }
        }
      }
      n139 = Greater Or Equal?(x=w59, y=4e-10) -> (x >= y?=w130:bool)
      n140 = case shown="False" w130 {
        tunnel: w59 -> [w211 w231]
        tunnel: "hamaker\nconstant" -> [w210 w230]
        tunnel: "tip\nradius\nnm" -> [w208 w229]
        tunnel: "a0\nnm 2" -> [w209 _]
        tunnel: "effective\nmodulus\nPa" -> [w207 _]
        tunnel: [w206 w228] -> w137
        frame False {
          n141 = xnode "公式"("sep"=w211, "h"=w210, "a0"=w209, "r"=w208, "es"=w207) -> ("Result"=w206:dbl)  [unwired: 1 in, 1 out]
        }
        frame True {
          n142 = xnode "公式 2"("sep"=w231, "h"=w230, "r"=w229) -> ("Result"=w228:dbl)  [unwired: 1 in, 1 out]
        }
      }
      n143 = local read "spring constant\nN/m"() -> (w136:dbl)
      n144 = Divide(x=w137, y=w136) -> (x/y=w126:dbl)
      n145 = feedback #6 ("反馈节点")() -> (w125:dbl)
      n146 = feedback-in #6(w126) -> ()
      n147 = local read "invOLS\nm/V"() -> (w135:dbl)
      n148 = Divide(x=w125, y=w135) -> (x/y=w70:dbl)
      "defl voltage" <- w70
      n149 = feedback-in #1(w70) -> ()
      n150 = node(w72, path "C:/Users/90457/Desktop/OneDrive - National University of Singapore/RL AFM/labview-contact/Python RL/SAC 2/main_sac.py" ("module path"), "main" ("function name"), w71, dbl[] [], w95, w70, w74, w75, w79, w80) -> (w94:refnum<k35>, w68:errorcluster, →"return value":dbl[])  [unwired: 6 in, 2 out]
      n151 = Subtract(x=w100, y=w70) -> (x-y=→"error":dbl)
      "step loop" <- w64
    }
    n152 = Equal?(x=w32, y=w40) -> (x = y?=w44:bool)
    "ep loop" <- w40
  }
  n153 = property on="I" class="WFChart (strict)"("History Data"=dbl[] []) -> ()  [unwired: 2 in, 2 out]
  n154 = property on="P" class="WFChart (strict)"("History Data"=dbl[] []) -> ()  [unwired: 2 in, 2 out]
  n155 = local write "total step"(0 ("total step")) -> ()
  n156 = property on="ep reward" class="WFChart (strict)"("History Data"=dbl[] []) -> ()  [unwired: 2 in, 2 out]
  n157 = property on="loss_a" class="WFChart (strict)"("History Data"=dbl[] []) -> ()  [unwired: 2 in, 2 out]
  n158 = property on="loss_c" class="WFChart (strict)"("History Data"=dbl[] []) -> ()  [unwired: 2 in, 2 out]
  n159 = property on="ZVolt" class="WFChart (strict)"("History Data"=dbl[] []) -> ()  [unwired: 2 in, 2 out]
  n160 = Close Python Session(session in=w11, error in=w10) -> ()  [unwired: 1 out]
  "batch_size" <- "base batch number"
